vi "ArmSetHomeLEDs.vi"(1 "RedLEDDevRef":T1={"DIO Channel"=enum."Invalid", "DevStatus"={"status"=FALSE, "code"=0, "source"=""}}, 2 "arm homing state":T4, 3 "YellowLEDDevRef":T1={"DIO Channel"=enum."Invalid", "DevStatus"={"status"=FALSE, "code"=0, "source"=""}}, 4 "GreenLEDDevRef":T1={"DIO Channel"=enum."Invalid", "DevStatus"={"status"=FALSE, "code"=0, "source"=""}}, 5 "Recovery":bool, 6 "arm homing validity":T3) -> ()   [LabVIEW 2018]
uses:
  TypeDefs/ArmHomingState.ctl
  TypeDefs/ArmHomingValidity.ctl
  <vilib>/Rock Robotics/WPI/DigitalOutput/WPI_DigitalOutputDevRef.ctl
  <vilib>/Rock Robotics/SystemInterfaces/DIO/FPGA_DIOChannel.ctl
  ArgosLib/IO/DIOLED/TypeDefs/DIOLEDMode.ctl
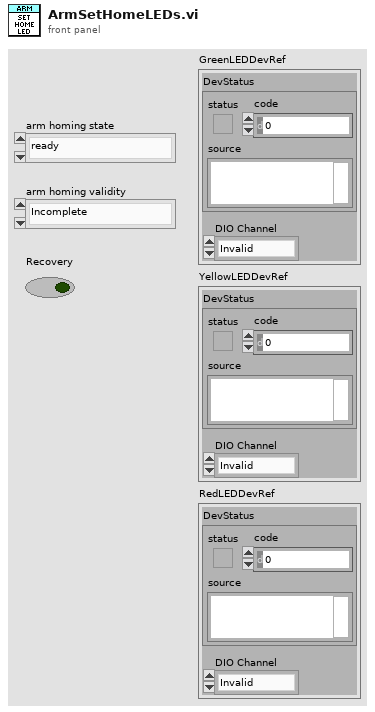
[diagram p1: front panel]
types:
  T1 = typedef "WPI_DigitalOutputDevRef.ctl" = cluster{"DIO Channel":T2, "DevStatus":errorcluster}
  T2 = typedef "FPGA_DIOChannel.ctl" = enum8{"DIO 0", "DIO 1", "DIO 2", "DIO 3", "DIO 4", "DIO 5", "DIO 6", "DIO 7", "DIO 8", "DIO 9", "DIO MXP 0", "DIO MXP 1", "DIO MXP 2", "DIO MXP 3", "DIO MXP 4", "DIO MXP 5", "DIO MXP 6", "DIO MXP 7", "DIO MXP 8", "DIO MXP 9", "DIO MXP 10", "DIO MXP 11", "DIO MXP 12", "DIO MXP 13", "DIO MXP 14", "DIO MXP 15", "SPI Port CS1", "SPI Port CS2", "SPI Port CS3", "SPI Port MISO", "SPI Port MOSI", "Invalid"}
  T3 = typedef "ArmHomingValidity.ctl" = enum16{"Incomplete", "Valid", "Invalid"}
  T4 = typedef "ArmHomingState.ctl" = enum16{"ready", "homing in progress", "homing complete ", "homing failed"}
  T5 = typedef "DIOLEDMode.ctl" = enum16{"Off", "On", "FastBlink", "SlowBlink"}
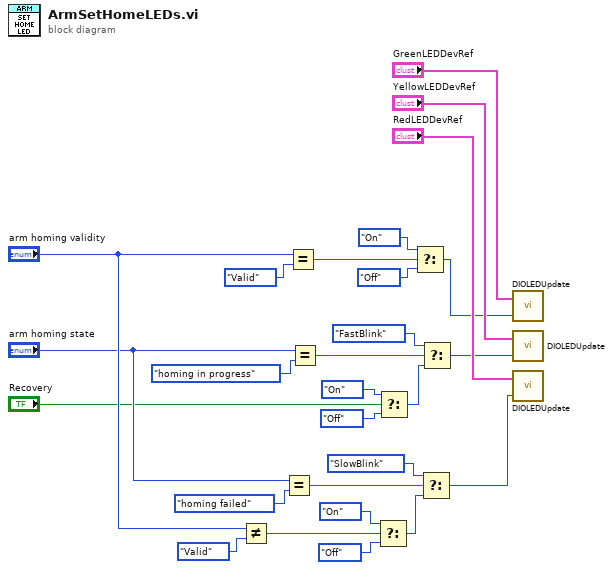
[diagram p0: block diagram]
diagram:
  n1 = Not Equal?(x="arm homing validity", y=ArmHomingValidity."Valid") -> (x != y?=w9:bool)
  n2 = Equal?(x="arm homing state", y=ArmHomingState."homing failed") -> (x = y?=w6:bool)
  n3 = Equal?(x="arm homing validity", y=ArmHomingValidity."Valid") -> (x = y?=w19:bool)
  n4 = Equal?(x="arm homing state", y=ArmHomingState."homing in progress") -> (x = y?=w23:bool)
  n5 = Select(t=DIOLEDMode."On" ("DIO LED Mode"), s=w9, f=DIOLEDMode."Off") -> (s? t:f=w12:T5)
  n6 = Select(t=DIOLEDMode."On" ("DIO LED Mode"), s="Recovery", f=DIOLEDMode."Off") -> (s? t:f=w4:T5)
  n7 = Select(t=DIOLEDMode."On" ("DIO LED Mode"), s=w19, f=DIOLEDMode."Off") -> (s? t:f=w16:T5)
  n8 = Select(t=DIOLEDMode."SlowBlink" ("DIO LED Mode"), s=w6, f=w12) -> (s? t:f=w11:T5)
  n9 = Select(t=DIOLEDMode."FastBlink" ("DIO LED Mode"), s=w23, f=w4) -> (s? t:f=w21:T5)
  n10 = call "DIOLEDUpdate.vi"("DIO LED Mode"=w16, "DIOLEDDevRefIn"="GreenLEDDevRef") -> ()  [unwired: 1 in, 1 out]
  n11 = call "DIOLEDUpdate.vi"("DIO LED Mode"=w21, "DIOLEDDevRefIn"="YellowLEDDevRef") -> ()  [unwired: 1 in, 1 out]
  n12 = call "DIOLEDUpdate.vi"("DIO LED Mode"=w11, "DIOLEDDevRefIn"="RedLEDDevRef") -> ()  [unwired: 1 in, 1 out]
